vi "Init Camera.vi"(8 "error in (no error)":errorcluster, 10 "Physical Camera Assignment":T1[](array[typedef]), 11 "Andor Camera in":refnum<class "Andor Camera.lvclass">) -> (0 "error out":errorcluster, 3 "Andor Camera out":refnum<class "Andor Camera.lvclass">)   [LabVIEW 2018, in "Andor Camera.lvlib" / "Andor Camera.lvclass"]
uses:
  Andor Camera.lvclass
  Resources/Type Defs/Physical Camera Assignment.ctl
  <userlib>/atmcd64d.llb/FanMode_mode typedef.ctl
  <userlib>/atmcd64d.llb/HSSpeed_type typedef.ctl
  <userlib>/atmcd64d.llb/Shutter_type typedef.ctl
  <userlib>/atmcd64d.llb/Shutter_mode typedef.ctl
  <userlib>/atmcd64d.llb/EMGainMode_mode typedef.ctl
  Andor Camera.lvclass/Andor Camera.ctl
  Resources/GLOBAL/GLOBAL Time-critical.vi
  Camera/Camera.lvclass
panel:
  in  "temperature":i32=-60
  out "model":string
  out "Controller Card Model":string
  out "speed (MHz)":sgl format="%.2f"
  out "VS speed (us)":sgl format="%.2f"
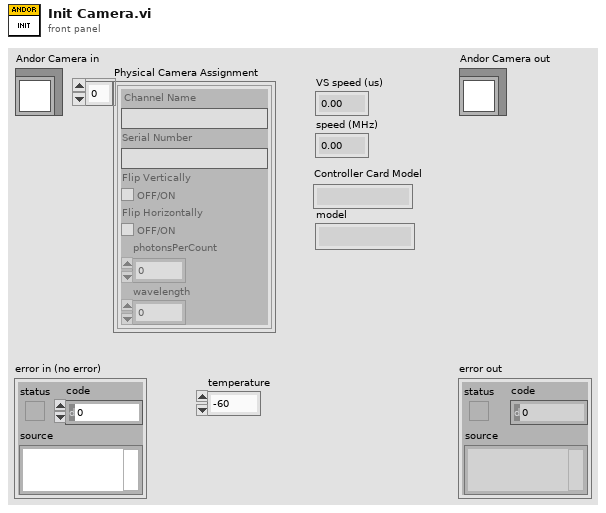
[diagram p1: front panel]
types:
  T1 = typedef "Physical Camera Assignment.ctl" = cluster{"Channel Name":string, "Serial Number":string, "Flip Vertically":bool, "Flip Horizontally":bool, "photonsPerCount":dbl, "wavelength":i16}
  T2 = typedef "EMGainMode_mode typedef.ctl" = enum16{"8-bit", "12-bit", "Linear", "Real"}
  T3 = typedef "FanMode_mode typedef.ctl" = enum16{"fan on full", "fan on low", "fan off"}
  T4 = typedef "Shutter_mode typedef.ctl" = enum16{"Auto", "Open", "Close", "N/A (3)", "Open FVB Series", "Open Any Series"}
  T5 = typedef "Shutter_type typedef.ctl" = enum16{"TTL Low", "TTL High"}
  T6 = typedef "HSSpeed_type typedef.ctl" = enum16{"EM Amp", "Conventional Amp"}
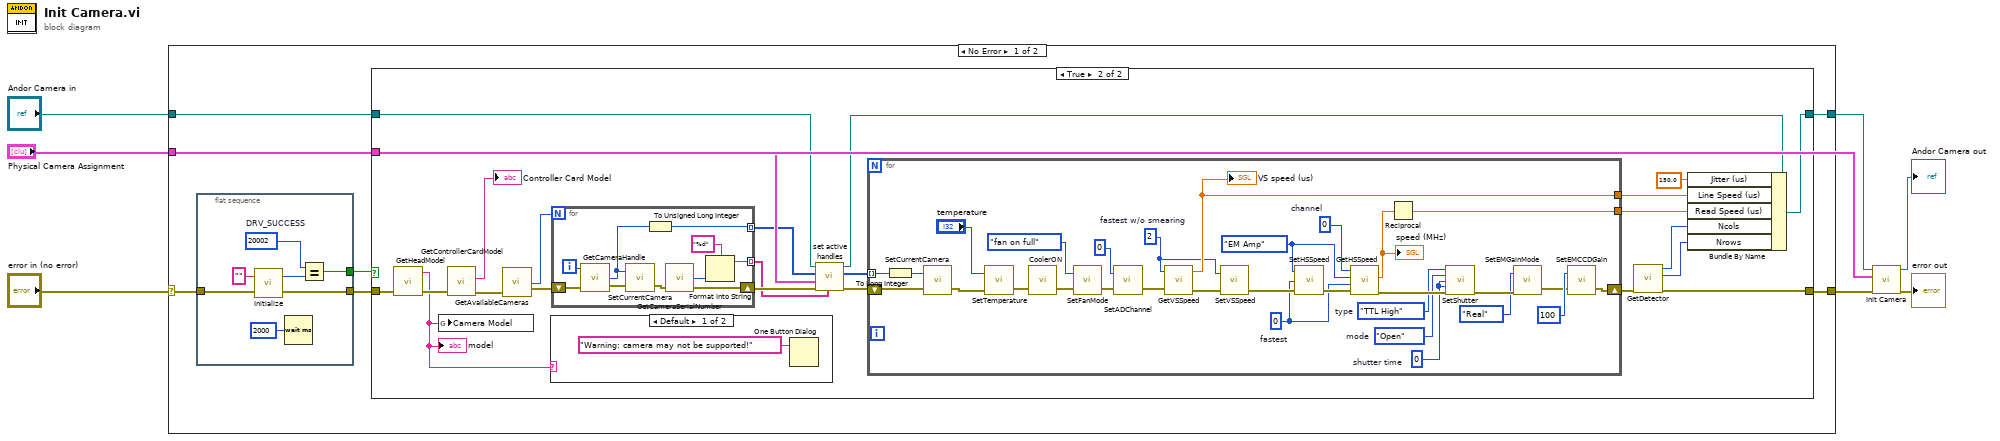
[diagram p0: block diagram]
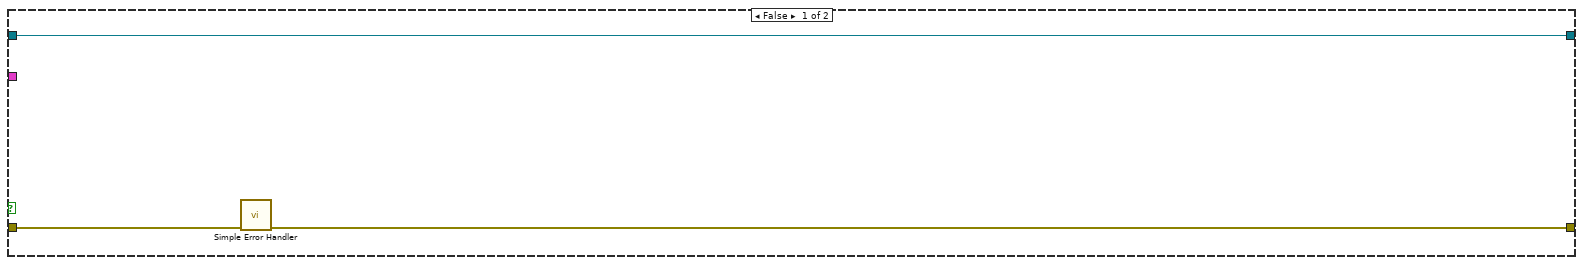
[diagram p2: hidden frame]
diagram:
  n1 = case shown="No Error" "error in (no error)" {
    selector: "error in (no error)" -> [w14 w90]
    tunnel: [w13 w90] -> w4
    tunnel: "Physical Camera Assignment" -> [w9 _]
    tunnel: "Andor Camera in" -> [w11 w89]
    tunnel: [w10 w89] -> w1
    frame No Error {
      n2 = flat-sequence {
        tunnel: w14 -> [w18]
        tunnel: [w17] -> w12
        tunnel: [w16] -> w8
        frame #0 {
          w19 = 20002  # DRV_SUCCESS
          n3 = call <userlib>:"Initialize.vi"("error in (no error)"=w18, "directory (\"\")"="" ("directory (\"\")")) -> ("error out"=w17:errorcluster, "DLL error code"=w20:u32)
          n4 = Wait (ms)(milliseconds to wait=u32 2000) -> ()  [unwired: 1 out]
          n5 = Equal?(x=w19, y=w20) -> (x = y?=w16:bool)
        }
      }
      n6 = case shown="True" w8 {
        tunnel: [w22 w42] -> w13
        tunnel: w12 -> [w23 w37]
        tunnel: w11 -> [w24 w31]
        tunnel: [w24 w47] -> w10
        tunnel: w9 -> [_ w27]
        frame False {
          n7 = call <vilib>:"Simple Error Handler.vi"("error in (no error)"=w23) -> ("error out"=w22:errorcluster)  [unwired: 4 in, 4 out]
        }
        frame True {
          n8 = call <userlib>:"GetHeadModel.vi"("error in (no error)"=w37) -> ("error out"=w39:errorcluster, "model"=w25:string)  [unwired: 2 in, 1 out]
          "model" <- w25
          n9 = global write "GLOBAL Time-critical.vi" "Camera Model"(w25) -> ()
          n10 = call <userlib>:"GetControllerCardModel.vi"("error in (no error)"=w39) -> ("error out"=w36:errorcluster, "Controller Card Model"=→"Controller Card Model":string)  [unwired: 4 in, 1 out]
          n11 = call <userlib>:"GetAvailableCameras.vi"("error in (no error)"=w36) -> ("error out"=w35:errorcluster, "totalCameras"=w34:i32)  [unwired: 2 in, 1 out]
          n12 = case shown="Default" w25 {
            frame Default {
              n13 = One Button Dialog(message="Warning: camera may not be supported!") -> ()  [unwired: 1 in, 1 out]
            }
            frame "DU897_BV" {
            }
          }
          n14 = for {
            N: w34 -> [_]
            shift-right: [w56] -> w33
            shift-left: w35 -> [w55]
            tunnel: [w52] -> w28 mode=indexing
            tunnel: [w49] -> w26 mode=indexing
            i -> [w54]
            n15 = call <userlib>:"GetCameraHandle.vi"("error in (no error)"=w55, "cameraIndex"=w54) -> ("error out"=w57:errorcluster, "cameraHandle"=w50:i32)  [unwired: 1 in, 1 out]
            n16 = call <userlib>:"SetCurrentCamera.vi"("error in (no error)"=w57, "cameraHandle"=w50) -> ("error out"=w58:errorcluster)  [unwired: 1 out]
            n17 = To Unsigned Long Integer(number=w50) -> (unsigned 32bit integer=w49:u32)
            n18 = call <userlib>:"GetCameraSerialNumber.vi"("error in (no error)"=w58) -> ("error out"=w56:errorcluster, "number"=w53:i32)  [unwired: 2 in, 1 out]
            n19 = Format Into String(format string="%d", w53) -> (resulting string=w52:string)  [unwired: 2 in, 1 out]
          }
          n20 = call-dynamic "set active handles.vi"("serial numbers"=w28, "error in (no error)"=w33, "All Camera"=w27, "All Handles"=w26, "Camera in"=w31) -> ("error out"=w32:errorcluster, "Selected Handles"=w29:u32[], "Camera out"=w30:refnum<class "Andor Camera.lvclass">)  [unwired: 3 in, 1 out]
          n21 = for {
            tunnel: [w88] -> w45
            tunnel: [w87] -> w44
            shift-right: [w86] -> w43
            shift-left: w32 -> [w62]
            tunnel: w29 -> [w60] mode=indexing
            w67 = 2  # fastest w/o smearing
            w72 = Shutter_mode_typedef."Open"  # mode
            w73 = Shutter_type_typedef."TTL High"  # type
            w74 = 0  # shutter time
            w77 = 0  # channel
            w78 = 0  # fastest
            w79 = HSSpeed_type_typedef."EM Amp" ("type")
            n22 = To Long Integer(number=w60) -> (32bit integer=w61:i32)
            n23 = call <userlib>:"SetCurrentCamera.vi"("error in (no error)"=w62, "cameraHandle"=w61) -> ("error out"=w59:errorcluster)  [unwired: 1 out]
            n24 = call <userlib>:"SetTemperature.vi"("error in (no error)"=w59, "temperature"="temperature") -> ("error out"=w85:errorcluster)  [unwired: 1 out]
            n25 = call <userlib>:"CoolerON.vi"("error in (no error)"=w85) -> ("error out"=w82:errorcluster)  [unwired: 1 in, 1 out]
            n26 = call <userlib>:"SetFanMode.vi"("error in (no error)"=w82, "mode"=FanMode_mode_typedef."fan on full") -> ("error out"=w70:errorcluster)  [unwired: 1 out]
            n27 = call <userlib>:"SetADChannel.vi"("error in (no error)"=w70, "channel"=0) -> ("error out"=w69:errorcluster)  [unwired: 1 out]
            n28 = call <userlib>:"GetVSSpeed.vi"("error in (no error)"=w69, "index"=w67) -> ("error out"=w68:errorcluster, "speed"=w87:sgl)  [unwired: 1 in, 1 out]
            "VS speed (us)" <- w87
            n29 = call <userlib>:"SetVSSpeed.vi"("error in (no error)"=w68, "index"=w67) -> ("error out"=w80:errorcluster)  [unwired: 1 out]
            n30 = call <userlib>:"SetHSSpeed.vi"("error in (no error)"=w80, "index"=w78, "type"=w79) -> ("error out"=w81:errorcluster)  [unwired: 1 in, 1 out]
            n31 = call <userlib>:"GetHSSpeed.vi"("error in (no error)"=w81, "index"=w78, "type"=w79, "channel"=w77) -> ("error out"=w75:errorcluster, "speed"=w76:sgl)  [unwired: 1 in, 1 out]
            "speed (MHz)" <- w76
            n32 = Reciprocal(x=w76) -> (1/x=w88:sgl)
            n33 = call <userlib>:"SetShutter.vi"("type"=w73, "mode"=w72, "closingtime"=w74, "openingtime"=w74, "error in (no error)"=w75) -> ("error out"=w65:errorcluster)  [unwired: 9 in, 1 out]
            n34 = call <userlib>:"SetEMGainMode.vi"("error in (no error)"=w65, "mode"=EMGainMode_mode_typedef."Real") -> ("error out"=w64:errorcluster)  [unwired: 1 out]
            n35 = call <userlib>:"SetEMCCDGain.vi"("error in (no error)"=w64, "gain"=100) -> ("error out"=w86:errorcluster)  [unwired: 1 out]
          }
          n36 = call <userlib>:"GetDetector.vi"("error in (no error)"=w43) -> ("error out"=w42:errorcluster, "ypixels"=w40:i32, "xpixels"=w41:i32)  [unwired: 3 in, 1 out]
          n37 = Bundle By Name(cluster=w30, "Jitter (us)"=150.0 ("Camera Timing.Jitter (us)"), "Line Speed (us)"=w44, "Read Speed (us)"=w45, "Ncols"=w41, "Nrows"=w40) -> (w47:refnum<class "Andor Camera.lvclass">)
        }
      }
    }
    frame Error {
    }
  }
  n38 = call-parent "Init Camera.vi"("error in (no error)"=w4, "Physical Camera Assignment"="Physical Camera Assignment", "Camera in"=w1) -> ("error out"=→"error out":errorcluster, "Camera out"=→"Andor Camera out":refnum<class "Andor Camera.lvclass">)  [unwired: 7 in]
